vi "Main.vi"() -> ()   [LabVIEW 2017]
doc: "The myRIO Project template acquires acceleration data from the onboard accelerometer and displays the changes of acceleration values in a waveform chart."
uses:
  <vilib>/myRIO/Common/Instrument Driver Framework/myRIO v1.0/Encoder/typedefs/Encoder Count Direction Enum.ctl
  Motor Status Enum.ctl
  <vilib>/myRIO/Instrument Drivers/Onboard IO/PWM/typedefs/PWM Reference.ctl
  <vilib>/myRIO/Common/Instrument Driver Framework/Utilities/typedefs/myRIO Generic Hardware Reference.ctl
  <vilib>/myRIO/Common/Instrument Driver Framework/Utilities/typedefs/Hardware Version Enum.ctl
  <vilib>/myRIO/Common/Instrument Driver Framework/Utilities/typedefs/myRIO v1.0 Reference.ctl
  <vilib>/myRIO/Common/Instrument Driver Framework/Utilities/typedefs/Generic FPGA Reference.ctl
  <vilib>/myRIO/Common/Instrument Driver Framework/myRIO v1.0/PWM/typedefs/PWM Channels Enum.ctl
  <vilib>/myRIO/Instrument Drivers/Onboard IO/PWM/typedefs/PWM Configuration.ctl
  <vilib>/userdefined/High Color/nirio_resource_hc.ctl
  <vilib>/myRIO/Common/Instrument Driver Framework/Utilities/vis/Is FPGA Ref Available.vi
  <vilib>/myRIO/Common/Instrument Driver Framework/myRIO v1.0/PWM/vis/myRIO v1.1 Open PWM.vi
  <vilib>/myRIO/Instrument Drivers/Onboard IO/PWM/vis/Set Duty Cycle and Frequency.vi
  <vilib>/myRIO/Common/Instrument Driver Framework/Utilities/vis/Validate Channels.vi
  <vilib>/myRIO/Common/Instrument Driver Framework/myRIO v1.0/PWM/vis/myRIO v1.0 Reserve PWM.vi
  <vilib>/myRIO/Common/Instrument Driver Framework/myRIO v1.0/UART/vis/myRIO v1.0 Close UART.vi
  <vilib>/myRIO/Common/Instrument Driver Framework/myRIO v1.0/PWM/vis/myRIO v1.0 Build MUX Configuration PWM.vi
  <vilib>/myRIO/Common/Instrument Driver Framework/myRIO v1.0/Resource Manager/vis/myRIO v1.0 Reserve Channel List.vi
  <vilib>/myRIO/Common/Instrument Driver Framework/myRIO v1.0/Resource Manager/vis/myRIO v1.0 Create Configuration List.vi
  <vilib>/myRIO/Common/Instrument Driver Framework/myRIO v1.0/Resource Manager/vis/myRIO v1.0 Reserve Channel.vi
  <vilib>/myRIO/Common/Instrument Driver Framework/myRIO v1.0/Resource Manager/vis/myRIO v1.0 Unreserve Channel.vi
  <vilib>/myRIO/Common/Instrument Driver Framework/myRIO v1.0/Resource Manager/vis/myRIO v1.0 Build Mutex Name.vi
  <vilib>/Utility/VariantDataType/GetNumericInfo.vi
  <vilib>/Utility/error.llb/Error Cluster From Error Code.vi
  <vilib>/myRIO/Common/Instrument Driver Framework/myRIO v1.0/myRIO v1.1 Open.vi
  <vilib>/myRIO/Common/Instrument Driver Framework/Utilities/vis/IO Manager.vi
  <vilib>/myRIO/Common/Instrument Driver Framework/Utilities/vis/Configuration Manager.vi
  <vilib>/myRIO/Common/Instrument Driver Framework/myRIO v1.0/Resource Manager/vis/myRIO v1.0 Configure IO.vi
  <vilib>/myRIO/Common/Instrument Driver Framework/myRIO v1.0/myRIO v1.0 Close.vi
  <vilib>/myRIO/Common/Instrument Driver Framework/myRIO v1.0/PWM/vis/myRIO v1.0 Write PWM.vi
  <vilib>/myRIO/Common/Instrument Driver Framework/Utilities/vis/FPGA Ref Manager.vi
  <vilib>/myRIO/Common/Instrument Driver Framework/myRIO v1.0/myRIO v1.0 Reset FPGA.vi
  <vilib>/myRIO/Common/Instrument Driver Framework/myRIO v1.0/IRQ/vis/myRIO v1.0 IRQ Info FGV.vi
  <vilib>/myRIO/Common/Instrument Driver Framework/myRIO v1.0/IRQ/vis/myRIO v1.0 Timer IRQ Info FGV.vi
  <vilib>/myRIO/Common/Instrument Driver Framework/myRIO v1.0/IRQ/vis/myRIO v1.0 ISR Agent.vi
  <vilib>/myRIO/Express VI/Onboard IO/PWM/PWM Express VI.xnode
  <vilib>/myRIO/Instrument Drivers/Onboard IO/PWM/vis/myRIO PWM Open.xnode
  <vilib>/myRIO/Instrument Drivers/Utilities/Utilities.lvlib
  <vilib>/myRIO/Instrument Drivers/Onboard IO/PWM/PWM.lvlib
panel:
  out "X Axis state":T1
  out "Y Axis state":T1
  out "Loop Runtime (s)":dbl format="%.3f"
  in  "Clear Chart History":bool
  in  "Coordinates Input":cluster{"X-axis (mm)":dbl, "Y-axis (mm)":dbl}
  out "Y Axis":T2(graph)
  out "X Axis":T2(graph)
  in  "X Axis Motor Target":T3
  out "X Axis Motor Params":T4
  in  "Y Axis Motor Target":T5
  out "Y Axis Motor Params":T5
  in  "stop":bool
  out "Output String":string
  out "Encoder Output":T7
  out "Total Runtime (s)":dbl format="%.2f"
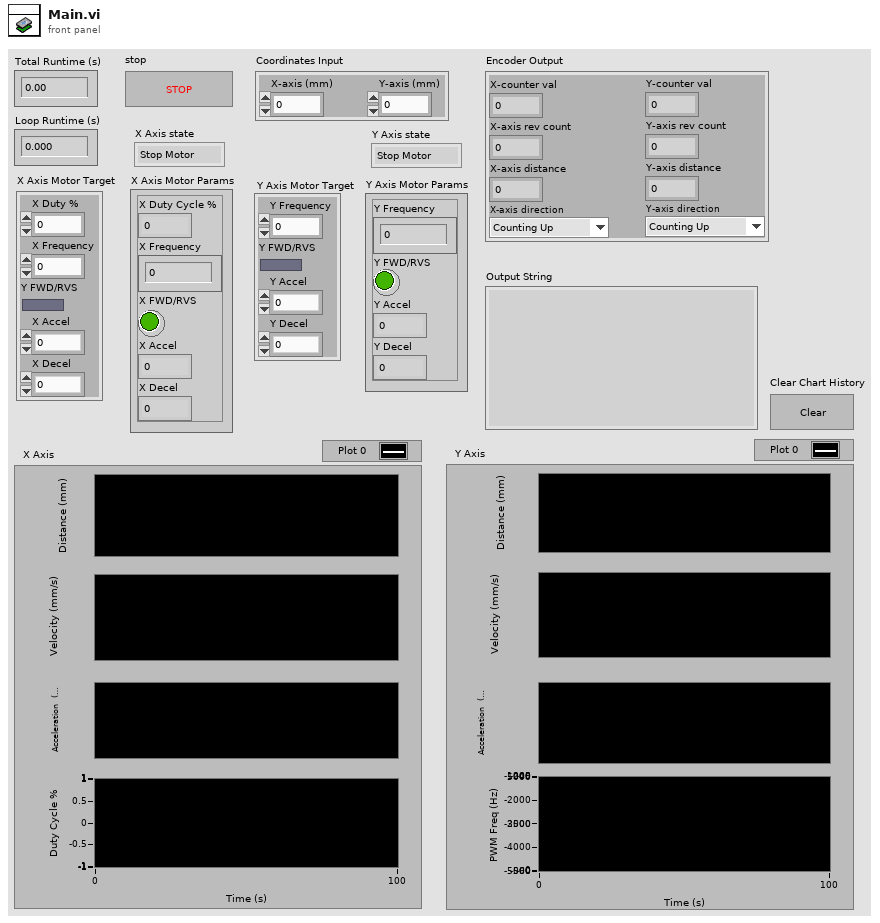
[diagram p1: front panel]
types:
  T1 = typedef "Motor Status Enum.ctl" = enum16{"Stop Motor", "Read Inputs", "Steady Speed", "Accelerate", "Decelerate"}
  T2 = cluster{"X-axis distance":dbl, dbl, dbl, "X Frequency":dbl}
  T3 = cluster{"X Frequency":dbl, "Y FWD/RVS":bool, "X Accel":dbl, "X Decel":dbl, "X Duty %":dbl}
  T4 = cluster{"X Frequency":dbl, "X FWD/RVS":bool, "X Accel":dbl, "X Decel":dbl, "X Duty Cycle %":dbl}
  T5 = cluster{"Y Frequency":dbl, "Y FWD/RVS":bool, "Y Accel":dbl, "Y Decel":dbl}
  T6 = typedef "Encoder Count Direction Enum.ctl" = enum16{"Counting Up", "Counting Down"}
  T7 = cluster{"Y-axis rev count":dbl, "Y-axis distance":dbl, "X-axis rev count":dbl, "X-axis distance":dbl, "Y-axis direction":T6, "X-axis direction":T6, "X-counter val":i32, "Y-counter val":i32}
  T8 = cluster{"X-axis distance":dbl, dbl, dbl, "X Frequency":dbl}[]
  T9 = cluster{dbl, dbl, "X-axis distance":dbl, "X Duty Cycle %":dbl, "X Frequency":dbl, "Y-axis distance":dbl, "Y Frequency":dbl, "X Accel":dbl, "X Decel":dbl, "Y Accel":dbl, "Y Decel":dbl, "X-axis (mm)":dbl, "Y-axis (mm)":dbl}
  T10 = cluster{"X-axis distance":dbl, dbl, dbl, "X Duty Cycle %":dbl}
  T11 = cluster{"Y-axis distance":dbl, dbl, dbl, "Y Frequency":dbl}
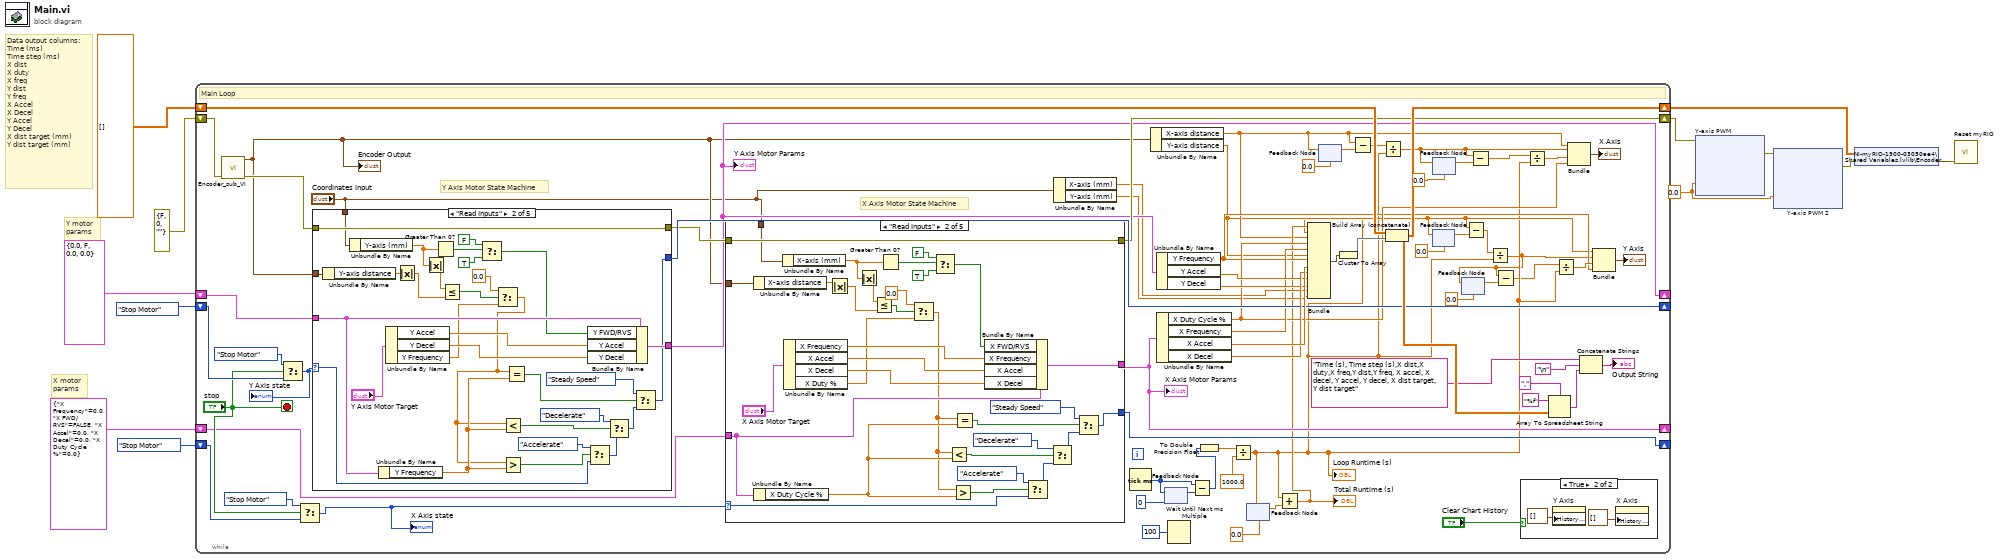
[diagram p0: block diagram]
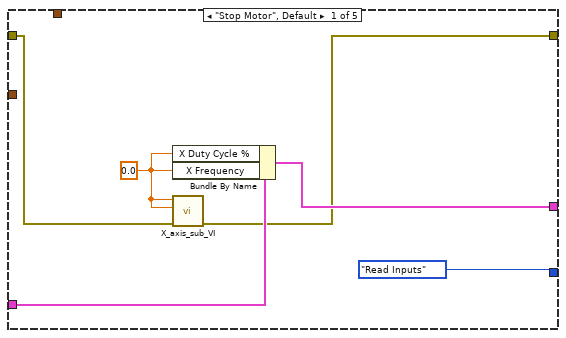
[diagram p3: hidden frame]
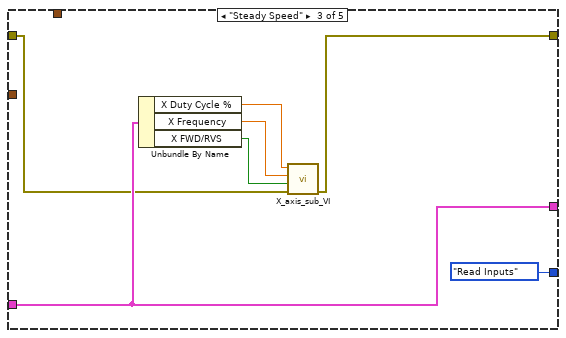
[diagram p4: hidden frame]
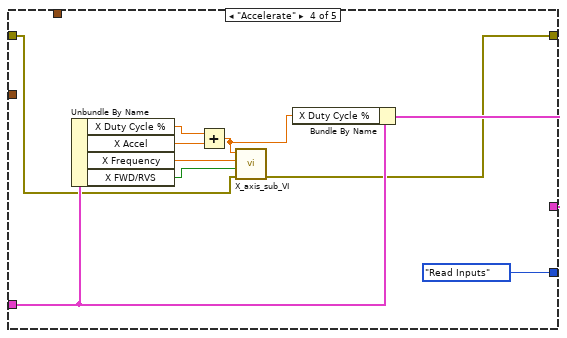
[diagram p5: hidden frame]
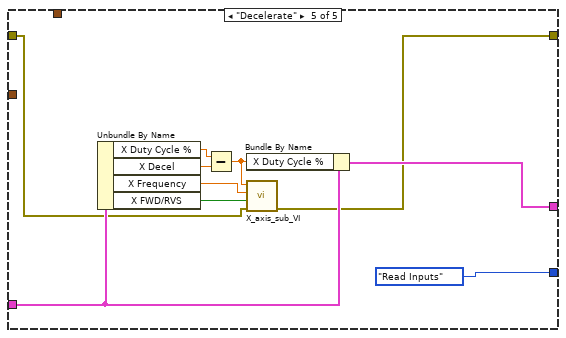
[diagram p6: hidden frame]
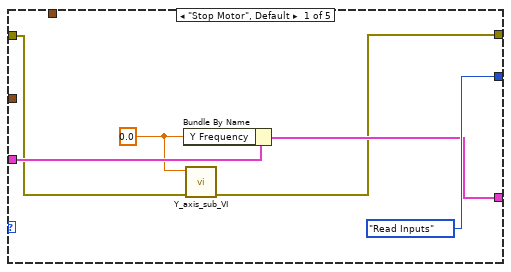
[diagram p7: hidden frame]
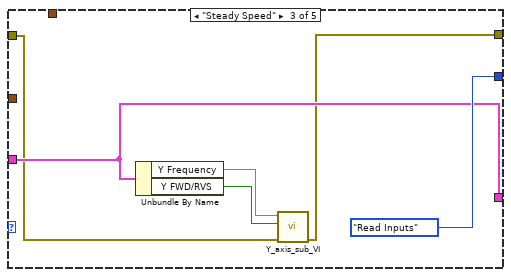
[diagram p8: hidden frame]
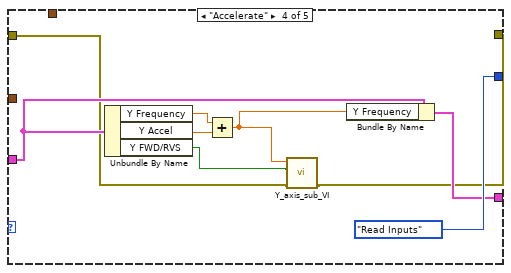
[diagram p9: hidden frame]
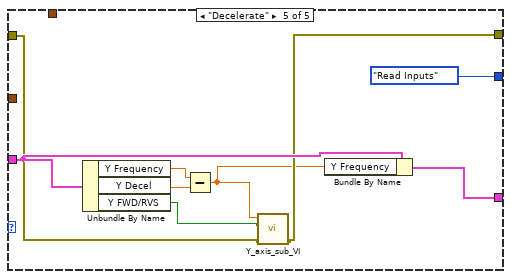
[diagram p10: hidden frame]
diagram:
  w5 = 0.0 ("Frequency [Hz]")
  # "X motor \nparams"
  # "Y motor \nparams"
  # "Data output columns:\nTime (ms)\nTime step (ms)\nX dist\nX duty\nX freq\nY dist\nY freq\nX Accel\nX Decel\nY Accel\nY Decel\nX dist target (mm)\nY dist target (mm)"
  n1 = while {
    shift-right: [w59] -> w12
    shift-left: errorcluster {"status"=FALSE, "code"=0, "source"=""} ("error in (no error)") -> [w82]
    shift-right: [w79] -> w8
    shift-left: dbl[][] [] -> [w78]
    shift-right: [w51] -> _
    shift-left: T5 {"Y Frequency"=0.0, "Y FWD/RVS"=FALSE, "Y Accel"=0.0, "Y Decel"=0.0} ("Y Axis Motor Params 2") -> [w72]
    shift-right: [w71] -> _
    shift-left: Motor_Status_Enum."Stop Motor" -> [w69]
    shift-right: [w62] -> _
    shift-left: Motor_Status_Enum."Stop Motor" -> [w64]
    shift-right: [w52] -> _
    shift-left: T4 {"X Frequency"=0.0, "X FWD/RVS"=FALSE, "X Accel"=0.0, "X Decel"=0.0, "X Duty Cycle %"=0.0} ("X Axis Motor Params 3") -> [w61]
    stop <- "stop" stop-if-true
    # "X Axis Motor State Machine"
    # "Y Axis Motor State Machine"
    # "Main Loop"
    n2 = call "Encoder_sub_VI.vi"("error in (no error)"=w82) -> ("error out"=w67:errorcluster, "Encoder Output"=w50:T7)  [unwired: 9 in]
    "Encoder Output" <- w50
    n3 = Select(t=Motor_Status_Enum."Stop Motor", s="stop", f=w69) -> (s? t:f=w70:T1)
    "Y Axis state" <- w70
    n4 = Select(t=Motor_Status_Enum."Stop Motor", s="stop", f=w64) -> (s? t:f=w65:T1)
    "X Axis state" <- w65
    n5 = case shown="\"Read Inputs\"" w70 {
      selector: w70 -> [_ w172 _ _ _]
      tunnel: w72 -> [w155 w173 w189 w198 w206]
      tunnel: [Motor_Status_Enum."Read Inputs" w156 Motor_Status_Enum."Read Inputs" Motor_Status_Enum."Read Inputs" Motor_Status_Enum."Read Inputs"] -> w71
      tunnel: [w153 w174 w189 w197 w207] -> w51
      tunnel: w67 -> [w151 w171 w188 w194 w204]
      tunnel: [w152 w171 w187 w193 w205] -> w60
      tunnel: w50 -> [_ w170 _ _ _]
      tunnel: "Coordinates Input" -> [_ w166 _ _ _]
      frame "Stop Motor", Default {
        w150 = 0.0 ("Y Frequency")
        n6 = Bundle By Name(cluster=w155, "Y Frequency"=w150) -> (w153:T5)
        n7 = call "Y_axis_sub_VI.vi"("error in (no error)"=w151, "Frequency"=w150) -> ("error out"=w152:errorcluster)  [unwired: 9 in]
      }
      frame "Read Inputs" {
        n8 = Unbundle By Name(w170) -> ("Y-axis distance"=w164:dbl)
        n9 = Unbundle By Name(w166) -> ("Y-axis (mm)"=w163:dbl)
        n10 = Unbundle By Name(w173) -> ("Y Frequency"=w180:dbl)
        n11 = Unbundle By Name("Y Axis Motor Target") -> ("Y Accel"=w184:dbl, "Y Decel"=w185:dbl, "Y Frequency"=w158:dbl)
        n12 = Absolute Value(x=w164) -> (abs(x)=w161:dbl)
        n13 = Absolute Value(x=w163) -> (abs(x)=w162:dbl)
        n14 = Greater Than 0?(x=w163) -> (x > 0?=w165:bool)
        n15 = Less Or Equal?(x=w162, y=w161) -> (x <= y?=w160:bool)
        n16 = Select(t=FALSE, s=w165, f=TRUE) -> (s? t:f=w167:bool)
        n17 = Select(t=0.0, s=w160, f=w158) -> (s? t:f=w157:dbl)
        n18 = Less?(x=w157, y=w180) -> (x < y?=w177:bool)
        n19 = Greater?(x=w157, y=w180) -> (0:w186:bool)
        n20 = Equal?(x=w157, y=w180) -> (x = y?=w181:bool)
        n21 = Bundle By Name(cluster=w173, "Y FWD/RVS"=w167, "Y Accel"=w184, "Y Decel"=w185) -> (w174:T5)
        n22 = Select(t=Motor_Status_Enum."Accelerate", s=w186, f=w172) -> (s? t:f=w179:T1)
        n23 = Select(t=Motor_Status_Enum."Decelerate", s=w177, f=w179) -> (s? t:f=w182:T1)
        n24 = Select(t=Motor_Status_Enum."Steady Speed", s=w181, f=w182) -> (s? t:f=w156:T1)
      }
      frame "Steady Speed" {
        n25 = Unbundle By Name(w189) -> ("Y Frequency"=w191:dbl, "Y FWD/RVS"=w192:bool)
        n26 = call "Y_axis_sub_VI.vi"("error in (no error)"=w188, "FWD/RVS"=w192, "Frequency"=w191) -> ("error out"=w187:errorcluster)  [unwired: 8 in]
      }
      frame "Accelerate" {
        n27 = Unbundle By Name(w198) -> ("Y Frequency"=w200:dbl, "Y Accel"=w201:dbl, "Y FWD/RVS"=w195:bool)
        n28 = Add(x=w200, y=w201) -> (x+y=w196:dbl)
        n29 = call "Y_axis_sub_VI.vi"("error in (no error)"=w194, "FWD/RVS"=w195, "Frequency"=w196) -> ("error out"=w193:errorcluster)  [unwired: 8 in]
        n30 = Bundle By Name(cluster=w198, "Y Frequency"=w196) -> (w197:T5)
      }
      frame "Decelerate" {
        n31 = Unbundle By Name(w206) -> ("Y Frequency"=w210:dbl, "Y Decel"=w209:dbl, "Y FWD/RVS"=w203:bool)
        n32 = Subtract(x=w210, y=w209) -> (x-y=w202:dbl)
        n33 = call "Y_axis_sub_VI.vi"("error in (no error)"=w204, "FWD/RVS"=w203, "Frequency"=w202) -> ("error out"=w205:errorcluster)  [unwired: 8 in]
        n34 = Bundle By Name(cluster=w206, "Y Frequency"=w202) -> (w207:T5)
      }
    }
    "Y Axis Motor Params" <- w51
    n35 = case shown="\"Read Inputs\"" w65 {
      selector: w65 -> [_ w110 _ _ _]
      tunnel: [Motor_Status_Enum."Read Inputs" w103 Motor_Status_Enum."Read Inputs" Motor_Status_Enum."Read Inputs" Motor_Status_Enum."Read Inputs"] -> w62
      tunnel: [w87 w109 w126 w133 w143] -> w52
      tunnel: w61 -> [w88 w108 w126 w132 w142]
      tunnel: w60 -> [w86 w106 w124 w131 w141]
      tunnel: [w85 w106 w123 w130 w140] -> w59
      tunnel: w50 -> [_ w105 _ _ _]
      tunnel: "Coordinates Input" -> [_ w104 _ _ _]
      frame "Stop Motor", Default {
        w90 = 0.0 ("Y Frequency")
        n36 = Bundle By Name(cluster=w88, "X Duty Cycle %"=w90, "X Frequency"=w90) -> (w87:T4)
        n37 = call "X_axis_sub_VI.vi"("error in (no error)"=w86, "Frequency"=w90, "Duty Cycle %"=w90) -> ("error out"=w85:errorcluster)  [unwired: 8 in]
      }
      frame "Read Inputs" {
        n38 = Unbundle By Name(w105) -> ("X-axis distance"=w97:dbl)
        n39 = Unbundle By Name(w108) -> ("X Duty Cycle %"=w121:dbl)
        n40 = Unbundle By Name(w104) -> ("X-axis (mm)"=w95:dbl)
        n41 = Unbundle By Name("X Axis Motor Target") -> ("X Frequency"=w113:dbl, "X Accel"=w111:dbl, "X Decel"=w112:dbl, "X Duty %"=w93:dbl)
        n42 = Absolute Value(x=w97) -> (abs(x)=w96:dbl)
        n43 = Absolute Value(x=w95) -> (abs(x)=w100:dbl)
        n44 = Less Or Equal?(x=w100, y=w96) -> (x <= y?=w99:bool)
        n45 = Greater Than 0?(x=w95) -> (x > 0?=w101:bool)
        n46 = Select(t=0.0, s=w99, f=w93) -> (s? t:f=w92:dbl)
        n47 = Select(t=FALSE, s=w101, f=TRUE) -> (s? t:f=w94:bool)
        n48 = Less?(x=w92, y=w121) -> (x < y?=w116:bool)
        n49 = Greater?(x=w92, y=w121) -> (0:w114:bool)
        n50 = Equal?(x=w92, y=w121) -> (x = y?=w120:bool)
        n51 = Bundle By Name(cluster=w108, "X FWD/RVS"=w94, "X Frequency"=w113, "X Accel"=w111, "X Decel"=w112) -> (w109:T4)
        n52 = Select(t=Motor_Status_Enum."Accelerate", s=w114, f=w110) -> (s? t:f=w118:T1)
        n53 = Select(t=Motor_Status_Enum."Decelerate", s=w116, f=w118) -> (s? t:f=w119:T1)
        n54 = Select(t=Motor_Status_Enum."Steady Speed", s=w120, f=w119) -> (s? t:f=w103:T1)
      }
      frame "Steady Speed" {
        n55 = Unbundle By Name(w126) -> ("X Duty Cycle %"=w128:dbl, "X Frequency"=w127:dbl, "X FWD/RVS"=w129:bool)
        n56 = call "X_axis_sub_VI.vi"("error in (no error)"=w124, "FWD/RVS"=w129, "Frequency"=w127, "Duty Cycle %"=w128) -> ("error out"=w123:errorcluster)  [unwired: 7 in]
      }
      frame "Accelerate" {
        n57 = Unbundle By Name(w132) -> ("X Duty Cycle %"=w135:dbl, "X Accel"=w136:dbl, "X Frequency"=w137:dbl, "X FWD/RVS"=w139:bool)
        n58 = Add(x=w135, y=w136) -> (x+y=w138:dbl)
        n59 = call "X_axis_sub_VI.vi"("error in (no error)"=w131, "FWD/RVS"=w139, "Frequency"=w137, "Duty Cycle %"=w138) -> ("error out"=w130:errorcluster)  [unwired: 7 in]
        n60 = Bundle By Name(cluster=w132, "X Duty Cycle %"=w138) -> (w133:T4)
      }
      frame "Decelerate" {
        n61 = Unbundle By Name(w142) -> ("X Duty Cycle %"=w145:dbl, "X Decel"=w146:dbl, "X Frequency"=w147:dbl, "X FWD/RVS"=w149:bool)
        n62 = Subtract(x=w145, y=w146) -> (x-y=w148:dbl)
        n63 = Bundle By Name(cluster=w142, "X Duty Cycle %"=w148) -> (w143:T4)
        n64 = call "X_axis_sub_VI.vi"("error in (no error)"=w141, "FWD/RVS"=w149, "Frequency"=w147, "Duty Cycle %"=w148) -> ("error out"=w140:errorcluster)  [unwired: 7 in]
      }
    }
    "X Axis Motor Params" <- w52
    n65 = Unbundle By Name("Coordinates Input") -> ("X-axis (mm)"=w36:dbl, "Y-axis (mm)"=w35:dbl)
    n66 = Tick Count (ms)() -> (millisecond timer value=w34:u32)
    n67 = Unbundle By Name(w50) -> ("X-axis distance"=w28:dbl, "Y-axis distance"=w18:dbl)
    n68 = Unbundle By Name(w51) -> ("Y Frequency"=w43:dbl, "Y Accel"=w75:dbl, "Y Decel"=w74:dbl)
    n69 = Unbundle By Name(w52) -> ("X Duty Cycle %"=w44:dbl, "X Frequency"=w47:dbl, "X Accel"=w77:dbl, "X Decel"=w76:dbl)
    n70 = feedback-in #1(w34) -> ()
    n71 = feedback #1(u32 0) -> (w33:u32)
    n72 = Wait Until Next ms Multiple(millisecond multiple=u32 100 ("milliseconds to wait")) -> ()  [unwired: 1 out]
    n73 = Subtract(x=w34, y=w33) -> (x-y=w40:u32)
    n74 = To Double Precision Float(number=w40) -> (double precision float=w38:dbl)
    n75 = Divide(x=w38, y=1000.0) -> (x/y=w17:dbl)
    "Loop Runtime (s)" <- w17
    n76 = feedback #2(0.0) -> (w31:dbl)
    n77 = feedback-in #2(w17) -> ()
    n78 = Add(x=w17, y=w31) -> (x+y=w30:dbl)
    "Total Runtime (s)" <- w30
    n79 = Bundle(w30, w17, "X-axis distance"=w28, "X Duty Cycle %"=w44, "X Frequency"=w47, "Y-axis distance"=w18, "Y Frequency"=w43, "X Accel"=w77, "X Decel"=w76, "Y Accel"=w75, "Y Decel"=w74, "X-axis (mm)"=w36, "Y-axis (mm)"=w35) -> (w80:T9)  [unwired: 1 in]
    n80 = feedback #3(0.0) -> (w27:dbl)
    n81 = feedback-in #3(w28) -> ()
    n82 = Cluster To Array(cluster=w80) -> (array=w81:dbl[])
    n83 = Subtract(x=w28, y=w27) -> (x-y=w26:dbl)
    n84 = Divide(x=w26, y=w17) -> (x/y=w23:dbl)
    n85 = Build Array (concatenate)(w78, w81) -> (w79:dbl[][])
    n86 = feedback #4(0.0) -> (w21:dbl)
    n87 = feedback-in #4(w18) -> ()
    n88 = feedback #5(0.0) -> (w25:dbl)
    n89 = feedback-in #5(w23) -> ()
    n90 = feedback #6(0.0) -> (w15:dbl)
    n91 = Subtract(x=w18, y=w21) -> (x-y=w19:dbl)
    n92 = Subtract(x=w23, y=w25) -> (x-y=w22:dbl)
    n93 = Divide(x=w19, y=w17) -> (x/y=w14:dbl)
    n94 = feedback-in #6(w14) -> ()
    n95 = Subtract(x=w14, y=w15) -> (x-y=w13:dbl)
    n96 = case shown="True" "Clear Chart History" {
      frame False {
      }
      frame True {
        n97 = property on="Y Axis" class="WFChart (strict)"("History Data"=T8 []) -> ()  [unwired: 2 in, 2 out]
        n98 = property on="X Axis" class="WFChart (strict)"("History Data"=T8 []) -> ()  [unwired: 2 in, 2 out]
      }
    }
    n99 = Divide(x=w22, y=w17) -> (x/y=w49:dbl)
    n100 = Array To Spreadsheet String(delimiter (Tab)=",", array=w79, 3:"%f" ("format string")) -> (spreadsheet string=w57:string)
    n101 = Divide(x=w13, y=w17) -> (x/y=w45:dbl)
    n102 = Bundle("X-axis distance"=w28, w23, w49, "X Duty Cycle %"=w44) -> (→"X Axis":T10)  [unwired: 1 in]
    n103 = Concatenate Strings("Time (s), Time step (s),X dist,X duty,X freq,Y dist,Y freq, X accel, X decel, Y accel, Y decel, X dist target, Y dist target", "\n", w57) -> (→"Output String":string)
    n104 = Bundle("Y-axis distance"=w18, w14, w45, "Y Frequency"=w43) -> (→"Y Axis":T11)  [unwired: 1 in]
  }
  n105 = xnode "Y-axis PWM"("Frequency [Hz]"=w5, "error in (no error)"=w12) -> ("error out"=w7:errorcluster)
  n106 = xnode "Y-axis PWM 2"("Frequency [Hz]"=w5, "error in (no error)"=w7) -> ("error out"=w6:errorcluster)
  n107 = shared-variable "NI-myRIO-1900-03050ae4\\Shared Variables.lvlib\\Encoder Data"(w8, error in=w6) -> (error out=w9:errorcluster)
  n108 = call <vilib>:"Reset myRIO.vi"("error in (no error)"=w9) -> ()  [unwired: 10 in, 1 out]
